vi "Actor Core.vi"(8 "error in":errorcluster, 11 "Generic Card in":refnum<class "Generic Card.lvclass">) -> (0 "error out":errorcluster, 3 "Actor out":refnum<class "Actor.lvclass">)   [LabVIEW 2014, in "Generic Instrument.lvlib" / "Generic Card.lvclass"]
doc: "(<B>Filename</B>: Actor Framework.lvlib:Actor.lvclass:Actor Core.vi)\n\nReceives messages to the actor, reacts to them, and initiates any error handling that may shut the actor down.\n\nDescendant classes may override this VI to append parallel tasks for the actor to complete while it handles messages. Overrides use the Call Parent Method node."
uses:
  Generic Card.lvclass
  <vilib>/ActorFramework/Actor/Actor.lvclass
  Generic Card.lvclass/Generic Card.ctl
  Display Panel/Abstract Display Messages/Write card number digit Msg/Write card number digit Msg.lvclass/Write card number digit Msg.ctl
  <vilib>/ActorFramework/Message Enqueuer/Message Enqueuer.lvclass/Message Enqueuer.ctl
  Generic Instrument.lvclass/Generic Instrument.ctl
  Display Panel/Abstract Display Messages/Write Instrument Name to Display Msg/Write Instrument Name to Display Msg.lvclass/Write Instrument Name to Display Msg.ctl
  <vilib>/ActorFramework/Message Enqueuer/Init from Existing Queue.vi
  <vilib>/ActorFramework/Message Enqueuer/Enqueue.vi
  <vilib>/ActorFramework/Message Priority Queue/Priority Enqueue.vi
  <vilib>/ActorFramework/Message Enqueuer/Message Enqueuer.lvclass
  Display Panel/Abstract Display Messages/Write card number digit Msg/Write card number digit Msg.lvclass
  Generic Instrument.lvclass
  Display Panel/Abstract Display Messages/Write Instrument Name to Display Msg/Write Instrument Name to Display Msg.lvclass
  <vilib>/MGI/Monitored Actor/Actor/Monitored Actor.lvclass
panel:
  out "Card #":u8
  out "Warm-Up Time":dbl
  # "Generic Card Class Core"
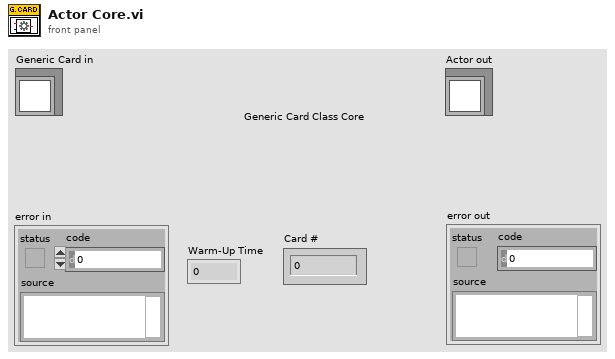
[diagram p1: front panel]
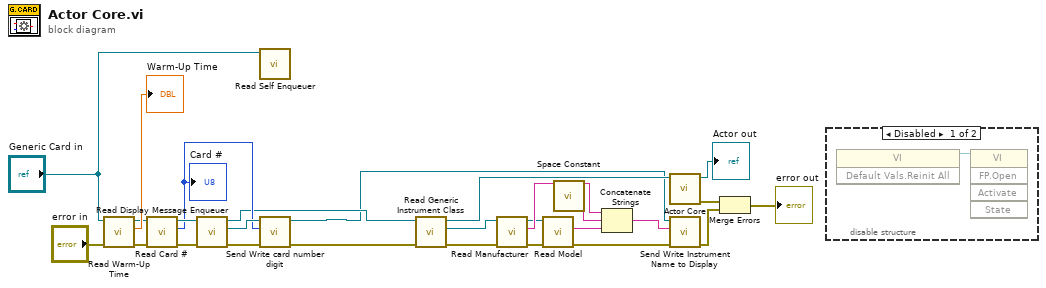
[diagram p0: block diagram]
diagram:
  n1 = call "Read Warm-Up Time.vi"("error in (no error)"="error in", "Generic Card in"="Generic Card in") -> ("error out"=w25:errorcluster, "Warm-Up Time"=→"Warm-Up Time":dbl, "Generic Card out"=w24:refnum<class "Generic Card.lvclass">)  [unwired: 7 in]
  n2 = call "Read Card #.vi"("error in (no error)"=w25, "Generic Card in"=w24) -> ("error out"=w18:errorcluster, "Card #"=w15:u8, "Generic Card out"=w19:refnum<class "Generic Card.lvclass">)  [unwired: 7 in]
  "Card #" <- w15
  n3 = call "Read Display Message Enqueuer.vi"("error in (no error)"=w18, "Generic Card in"=w19) -> ("error out"=w17:errorcluster, "Actor Framework.lvlib:Message Enqueuer"=w16:refnum<class "Message Enqueuer.lvclass">, "Generic Card out"=w14:refnum<class "Generic Card.lvclass">)  [unwired: 7 in]
  n4 = call <vilib>:"Read Self Enqueuer.vi"("Actor"="Generic Card in") -> ()  [unwired: 10 in, 1 out]
  n5 = call "Send Write card number digit.vi"("error in (no error)"=w17, "Card #"=w15, "Message Enqueuer"=w16) -> ("error out"=w1:errorcluster, "Message Enqueuer out"=w2:refnum<class "Message Enqueuer.lvclass">)  [unwired: 7 in]
  n6 = call "Read Generic Instrument Class.vi"("error in (no error)"=w1, "Generic Card in"=w14) -> ("error out"=w11:errorcluster, "Generic Instrument.lvlib:Generic Instrument.lvclass"=w12:refnum<class "Generic Instrument.lvclass">, "Generic Card out"=w13:refnum<class "Generic Card.lvclass">)  [unwired: 7 in]
  n7 = call "Read Manufacturer.vi"("error in (no error)"=w11, "Generic Instrument in"=w12) -> ("error out"=w6:errorcluster, "Manufacturer"=w10:string, "Generic Instrument out"=w8:refnum<class "Generic Instrument.lvclass">)  [unwired: 7 in]
  n8 = call "Read Model.vi"("error in (no error)"=w6, "Generic Instrument in"=w8) -> ("error out"=w5:errorcluster, "Model"=w7:string)  [unwired: 7 in, 1 out]
  n9 = call <vilib>:"Space Constant.vi"() -> ("String"=w9:string)
  n10 = Concatenate Strings(w10, w9, w7) -> (w4:string)
  n11 = call-parent "Actor Core.vi"("Actor in"=w13) -> ("error out"=w22:errorcluster, "Actor out"=→"Actor out":refnum<class "Actor.lvclass">)  [unwired: 9 in]
  n12 = call "Send Write Instrument Name to Display.vi"("error in (no error)"=w5, "Instrument Name"=w4, "Message Enqueuer"=w2) -> ("error out"=w3:errorcluster)  [unwired: 7 in, 1 out]
  n13 = Merge Errors(w22, w3) -> (→"error out":errorcluster)
  n14 = disable-structure shown="Disabled" {
    frame Disabled {
      n15 = invoke class="VI" method="Default Vals.Reinit All"() -> (reference out=w28:refnum<vi>)  [unwired: 3 in, 2 out]
      n16 = invoke class="VI" method="FP.Open"(reference=w28) -> ()  [unwired: 4 in, 5 out]
    }
    frame Enabled {
    }
  }
